vi "MethodVariantToPaths.vi"(1 "Method(s)":variant) -> (0 "Paths":path[](array[path]))   [LabVIEW 2014, in "LibReader.lvclass"]
uses:
  <resource>/Framework/Providers/Open_GDS/ClassProviders/LibProvider_BaseClassInterface/LibReader_class/LibReader.lvclass
  <resource>/Framework/Providers/Open_GDS/ClassProviders/Provider_BaseClassInterface/Types/ClassTypes_MethodType.ctl
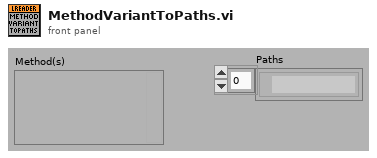
[diagram p1: front panel]
types:
  T1 = typedef "ClassTypes_MethodType.ctl" = cluster{"MethodName":string, "Visibility":enum16{"Public", "Private", "Protected"}, "StereoType":string, "Path":path}
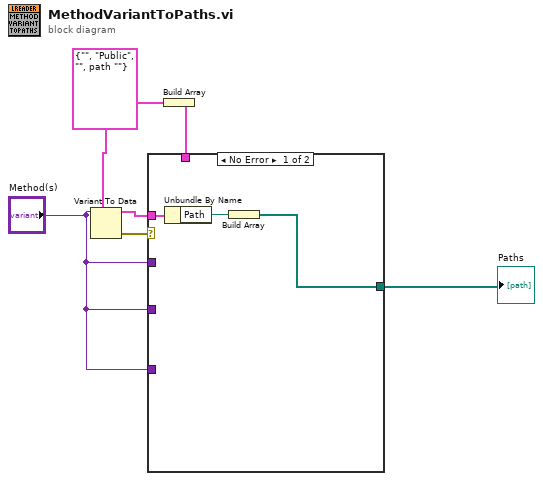
[diagram p0: block diagram]
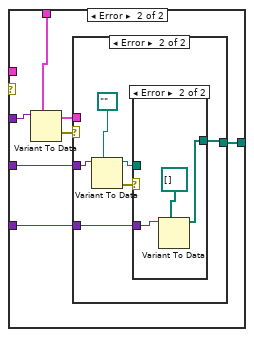
[diagram p2: hidden frame]
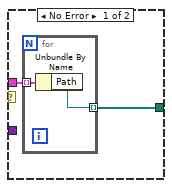
[diagram p3: hidden frame]
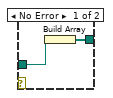
[diagram p4: hidden frame]
diagram:
  w4 = T1 {"MethodName"="", "Visibility"=enum."Public", "StereoType"="", "Path"=path ""} ("Method")
  n1 = Variant To Data(type=w4, Variant="Method(s)") -> (data=w2:T1, error out=w1:errorcluster)  [unwired: 1 in]
  n2 = Build Array(w4) -> (w5:T1[])
  n3 = case shown="No Error" w1 {
    tunnel: w2 -> [w9 _]
    tunnel: [w7 w12] -> w3
    tunnel: "Method(s)" -> [_ w16]
    tunnel: w5 -> [_ w15]
    tunnel: "Method(s)" -> [_ w11]
    tunnel: "Method(s)" -> [_ w10]
    frame No Error {
      n4 = Unbundle By Name(w9) -> ("Path"=w8:path)
      n5 = Build Array(w8) -> (w7:path[])
    }
    frame Error {
      n6 = Variant To Data(type=w15, Variant=w16) -> (data=w13:T1[], error out=w14:errorcluster)  [unwired: 1 in]
      n7 = case shown="Error" w14 {
        tunnel: w13 -> [w18 _]
        tunnel: [w17 w23] -> w12
        tunnel: w11 -> [_ w26]
        tunnel: w10 -> [_ w21]
        frame No Error {
          n8 = for {
            tunnel: w18 -> [w20] mode=indexing
            tunnel: [w19] -> w17 mode=indexing
            n9 = Unbundle By Name(w20) -> ("Path"=w19:path)
          }
        }
        frame Error {
          n10 = Variant To Data(type=path "" ("Path"), Variant=w26) -> (data=w22:path, error out=w24:errorcluster)  [unwired: 1 in]
          n11 = case shown="Error" w24 {
            tunnel: [w27 w29] -> w23
            tunnel: w22 -> [w28 _]
            tunnel: w21 -> [_ w31]
            frame No Error {
              n12 = Build Array(w28) -> (w27:path[])
            }
            frame Error {
              n13 = Variant To Data(type=path[] [], Variant=w31) -> (data=w29:path[])  [unwired: 1 in, 1 out]
            }
          }
        }
      }
    }
  }
  "Paths" <- w3
